vi "getShape.vi"(8 "error in (no error)":errorcluster, 10 "Shape":string, 11 "ShapeFactory in":refnum<class "ShapeFactory.lvclass">) -> (0 "error out":errorcluster, 2 "afShape.lvclass":refnum<class "afShape.lvclass">, 3 "ShapeFactory out":refnum<class "ShapeFactory.lvclass">)   [LabVIEW 2017, in "ShapeFactory.lvclass"]
uses:
  ShapeFactory.lvclass
  afShape Class/afShape.lvclass
  afCircle Class/afCircle.lvclass
  C:/Users/fflores/Documents/LabVIEW-Open-Projects/LabIVEW OOP Design Patterns/Abstract Factory Pattern/afShape Class/afShape.lvclass
  afRectangle Class/afRectangle.lvclass
  afSquare Class/afSquare.lvclass
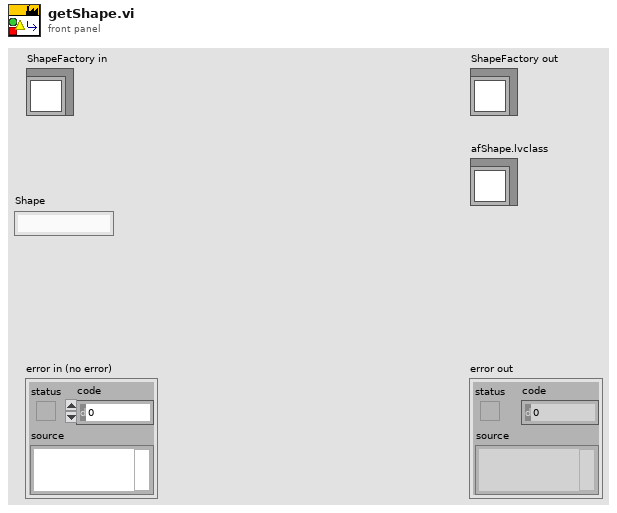
[diagram p1: front panel]
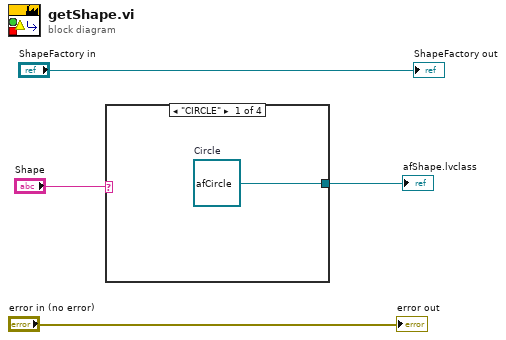
[diagram p0: block diagram]
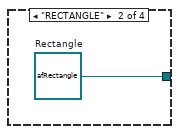
[diagram p2: hidden frame]
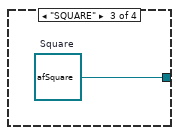
[diagram p3: hidden frame]
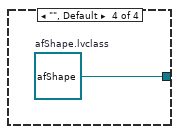
[diagram p4: hidden frame]
diagram:
  n1 = case shown="\"CIRCLE\"" "Shape" {
    tunnel: [w5 w6 w7 w8] -> w1
    frame "CIRCLE" {
      w5 = refnum<class "afCircle.lvclass"> refnum  # Circle
    }
    frame "RECTANGLE" {
      w6 = refnum<class "afRectangle.lvclass"> refnum  # Rectangle
    }
    frame "SQUARE" {
      w7 = refnum<class "afSquare.lvclass"> refnum  # Square
    }
    frame "", Default {
      w8 = refnum<class "afShape.lvclass"> refnum  # afShape.lvclass
    }
  }
  "afShape.lvclass" <- w1
  "error out" <- "error in (no error)"
  "ShapeFactory out" <- "ShapeFactory in"
